vi "ShotPos_FromShipPos.vi"() -> ()   [LabVIEW 2019]
panel:
  out "ShotPos":T1
  in  "ShipPos":T1
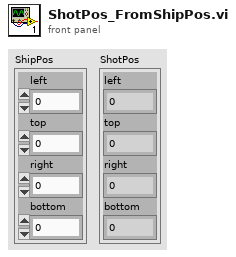
[diagram p1: front panel]
types:
  T1 = cluster{"left":i16, "top":i16, "right":i16, "bottom":i16}
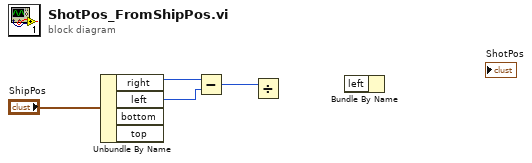
[diagram p0: block diagram]
diagram:
  n1 = Unbundle By Name("ShipPos") -> ("right"=w2:i16, "left"=w3:i16)  [unwired: 2 out]
  n2 = Subtract(x=w2, y=w3) -> (x-y=w1:i16)
  n3 = Divide(x=w1) -> ()  [unwired: 1 in, 1 out]
  n4 = Bundle By Name() -> ()  [unwired: 2 in, 1 out]
